vi "FFT Monitor.vi"() -> ()   [LabVIEW 2020]
uses:
  <vilib>/express/express analysis/Spectral/Block/exnSpectralBlock spectral measurements RMS poly.vi
  <vilib>/express/express analysis/Spectral/Block/exnSpectralBlock spectral measurements RMS DDT.vi
  <vilib>/express/express analysis/Spectral/XNode/ExpressSpectralMeasurementsBlockNode.xnode
panel:
  in  "stop":bool
  out "Waveform Graph":dynamicdata(graph)
  out "data":dynamicdata(graph)
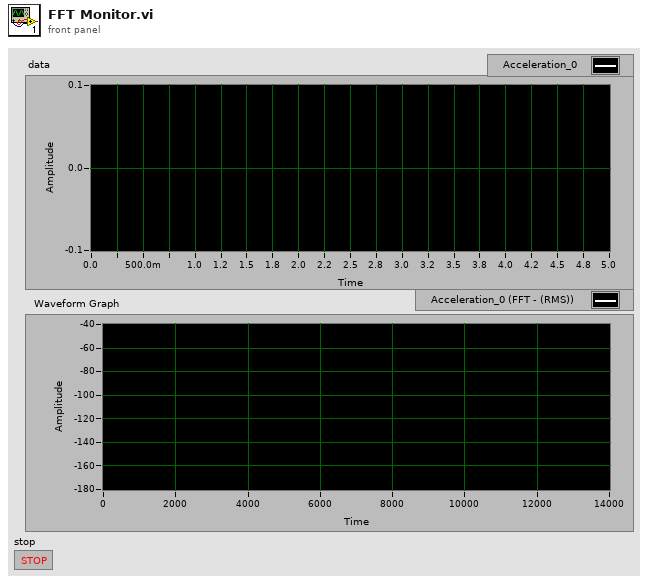
[diagram p1: front panel]
types:
  T1 = cluster{"averaging mode":u16, "weighting mode":u16, "number of averages":u32}
  T2 = cluster{"dB On (F)":bool, "unwrap phase (F)":bool, "convert to degree (F)":bool}
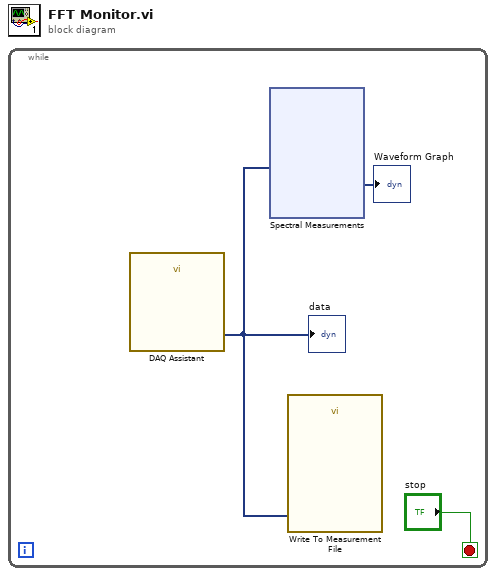
[diagram p0: block diagram]
diagram:
  n1 = while {
    stop <- "stop" stop-if-true
    n2 = call "DAQ Assistant"() -> ("data"=w2:dynamicdata)  [unwired: 17 in, 2 out]
    "data" <- w2
    n3 = xnode "Spectral Measurements"("Signals"=w2) -> ("FFT - (RMS)"=→"Waveform Graph":dynamicdata)  [unwired: 1 in, 2 out]
    n4 = call "Write To Measurement File"("Signals"=w2) -> ()  [unwired: 16 in, 3 out]
  }
